vi "Setup DCPower Current Sequence for ELOAD.vi"(7 "Channel Groups?":bool, 8 "error in (no error)":errorcluster, 9 "Parameters for Sequence":T1={"Supplies"=[], "Limit"=0.0, "Aperture Time"=0.0, "Settling Time"=0.0, "Sense"=1008, "Transient Response"=1041} {"Transient Response" items=["Slow"=1041, "Normal"=1038, "Fast"=1039, "Custom"=1042]; "Sense" items=["Local"=1008, "Remote"=1009]}, 10 "Channel List":string caption="channel name", 11 "DCPower Handle In":refnum<k15>) -> (0 "error out":errorcluster, 3 "DCPower Handle Out":refnum<k15>)   [LabVIEW 2021, in "PMIC Common.lvlib"]
uses:
  PMIC Common.lvlib
  <instrlib>/niDCPower/nidcpower.llb/niDCPower Source Mode.ctl
  <instrlib>/niDCPower/nidcpower.llb/niDCPower Output Function.ctl
  DCPower Parameters for Sequence.ctl
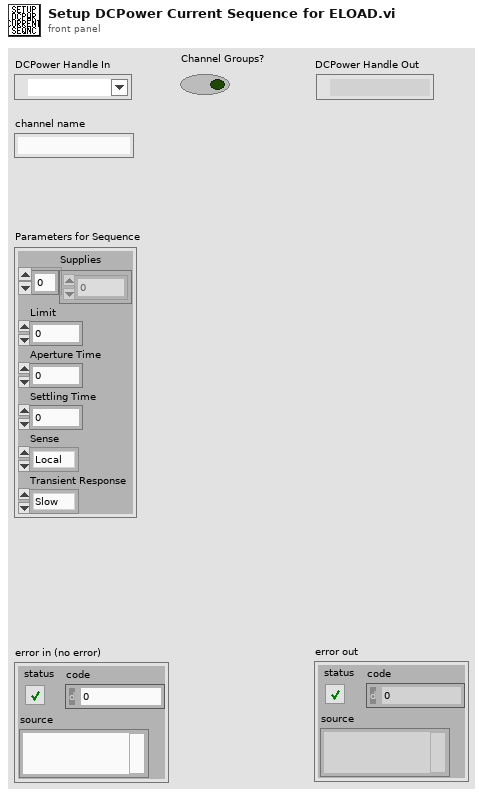
[diagram p1: front panel]
types:
  T1 = typedef "PMIC Common.lvlib/DCPower Parameters for Sequence.ctl" = cluster{"Supplies":dbl[], "Limit":dbl, "Aperture Time":dbl, "Settling Time":dbl, "Sense":i32, "Transient Response":i32}
  T2 = typedef "niDCPower Output Function.ctl" = i32
  T3 = typedef "niDCPower Source Mode.ctl" = i32
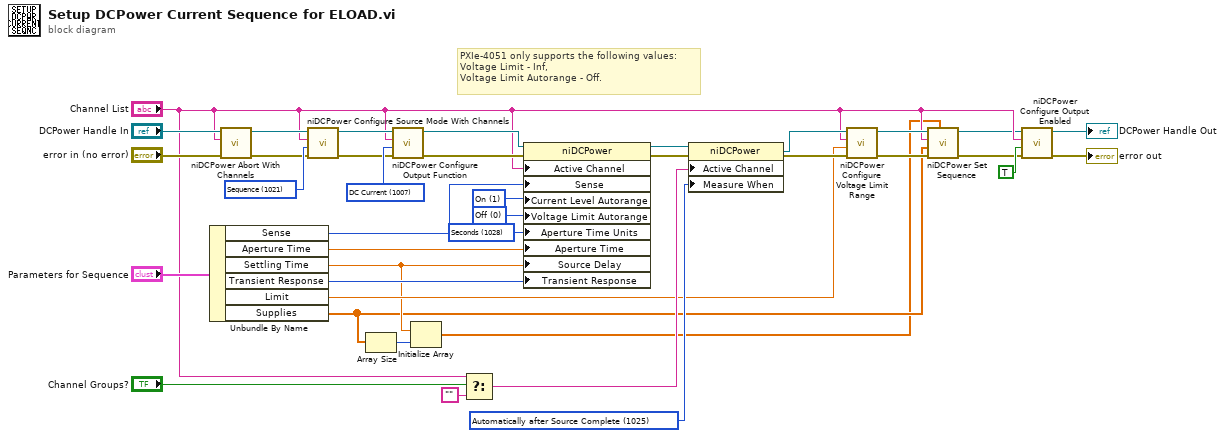
[diagram p0: block diagram]
diagram:
  w5 = 0 items=["Off", "On"] ("Source:DC Current:Voltage Limit Autorange")
  w20 = 1028 items=["Seconds"=1028, "Power Line Cycles"=1029] ("Measurement:Aperture Time Units")
  w22 = 1025 items=["Automatically after Source Complete"=1025, "On Demand"=1026, "On Measure Trigger"=1027] ("Measurement:Advanced:Measure When")
  w30 = 1 items=["Off", "On"] ("DC Voltage:Voltage Level Autorange")
  w34 = T2 1007 items=["DC Voltage"=1006, "DC Current"=1007, "Pulse Voltage"=1049, "Pulse Current"=1050] ("output function")
  w33 = T3 1021 items=["Single Point"=1020, "Sequence"=1021] ("source mode")
  # "PXIe-4051 only supports the following values:\nVoltage Limit - Inf,\nVoltage Limit Autorange - Off."
  n1 = Unbundle By Name("Parameters for Sequence") -> ("Sense"=w18:i32, "Aperture Time"=w17:dbl, "Settling Time"=w4:dbl, "Transient Response"=w16:i32, "Limit"=w11:dbl, "Supplies"=w2:dbl[])
  n2 = call <instrlib>:"niDCPower Abort With Channels.vi"("error in (no error)"="error in (no error)", "channel name"="Channel List", "instrument handle"="DCPower Handle In") -> ("error out"=w27:errorcluster, "instrument handle out"=w28:refnum<k15>)  [unwired: 7 in]
  n3 = call <instrlib>:"niDCPower Configure Source Mode With Channels.vi"("error in (no error)"=w27, "source mode"=w33, "channel name"="Channel List", "instrument handle"=w28) -> ("error out"=w31:errorcluster, "instrument handle out"=w32:refnum<k15>)  [unwired: 6 in]
  n4 = Array Size(array=w2) -> (size(s)=w3:i32)
  n5 = call <instrlib>:"niDCPower Configure Output Function.vi"("error in (no error)"=w31, "output function"=w34, "channel name"="Channel List", "instrument handle"=w32) -> ("error out"=w38:errorcluster, "instrument handle out"=w37:refnum<k15>)  [unwired: 6 out]
  n6 = Initialize Array(w4, w3) -> (w1:dbl[])
  n7 = Select(t="Channel List", s="Channel Groups?", f="") -> (s? t:f=w23:string)
  n8 = property class="niDCPower"(reference=w37, error in=w38, "Active Channel"="Channel List", "Sense"=w18, "Current Level Autorange"=w30, "Voltage Limit Autorange"=w5, "Aperture Time Units"=w20, "Aperture Time"=w17, "Source Delay"=w4, "Transient Response"=w16) -> (reference out=w35:refnum<k15>, error out=w36:errorcluster)
  n9 = property class="niDCPower"(reference=w35, error in=w36, "Active Channel"=w23, "Measure When"=w22) -> (reference out=w13:refnum<k15>, error out=w12:errorcluster)
  n10 = call <instrlib>:"niDCPower Configure Voltage Limit Range.vi"("error in (no error)"=w12, "voltage limit range"=w11, "channel name"="Channel List", "instrument handle"=w13) -> ("error out"=w9:errorcluster, "instrument handle out"=w10:refnum<k15>)  [unwired: 6 in]
  n11 = call <instrlib>:"niDCPower Set Sequence.vi"("source delays"=w1, "error in (no error)"=w9, "values"=w2, "channel name"="Channel List", "instrument handle"=w10) -> ("error out"=w6:errorcluster, "instrument handle out"=w7:refnum<k15>)  [unwired: 5 in]
  n12 = call <instrlib>:"niDCPower Configure Output Enabled.vi"("error in (no error)"=w6, "output enabled"=TRUE, "channel name"="Channel List", "instrument handle"=w7) -> ("error out"=→"error out":errorcluster, "instrument handle out"=→"DCPower Handle Out":refnum<k15>)  [unwired: 6 in]
